vi "Initial Values-Compare-STRING.vi"(5 "Function (Add)":T1=enum."Add", 7 "Current values":string[](array[string]), 8 "error in (no error)":errorcluster, 9 "Keys Array":T4, 10 "Section name":string, 11 "User profile ini file ref":T5) -> (0 "error out":errorcluster, 1 "Keys of changed parameters":T3, 2 "Changed parameters info":T2[](array[typedef]), 3 "User profile ini file ref":T5, 4 "Changes exist":bool)   [LabVIEW 2017]
uses:
  Typedefs/Ini file interface (String).ctl
  <vilib>/Utility/config.llb/Config Data RefNum.ctl
  User Interface/User profiles code/Typedefs/Changes info cluster-STRING.ctl
  User Interface/User profiles code/Typedefs/Changed parameter cluster.ctl
  User Interface/User profiles code/Typedefs/Comparison states.ctl
  <userlib>/_OpenG.lib/array/array.llb/Search 1D Array (Boolean)__ogtk.vi
  <userlib>/_OpenG.lib/array/array.llb/Index 1D Array Elements (String)__ogtk.vi
  <userlib>/_OpenG.lib/array/array.llb/Index 1D Array Elements (Variant)__ogtk.vi
  <vilib>/Utility/config.llb/NI_LVConfig.lvlib
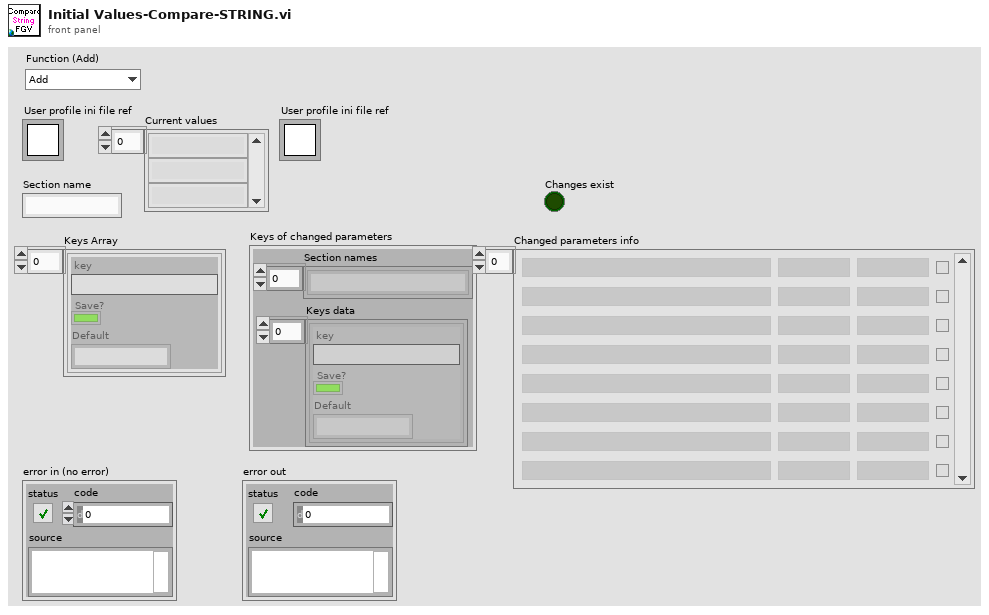
[diagram p1: front panel]
types:
  T1 = typedef "Comparison states.ctl" = enum16{"Init.", "Add", "Read"}
  T2 = typedef "Changed parameter cluster.ctl" = cluster{"Name":string, "Old value":string, "New value":string, "Save":bool}
  T3 = typedef "Changes info cluster-STRING.ctl" = cluster{"Section names":string[], "Keys data":T4}
  T4 = typedef "Ini file interface (String).ctl" = cluster{"key":string, "Save?":bool, "Default":string}[]
  T5 = typedef "NI_LVConfig.lvlib/Config Data RefNum.ctl" = refnum<k1>
  T6 = cluster{"key":string, "Save?":bool, "Default":string}
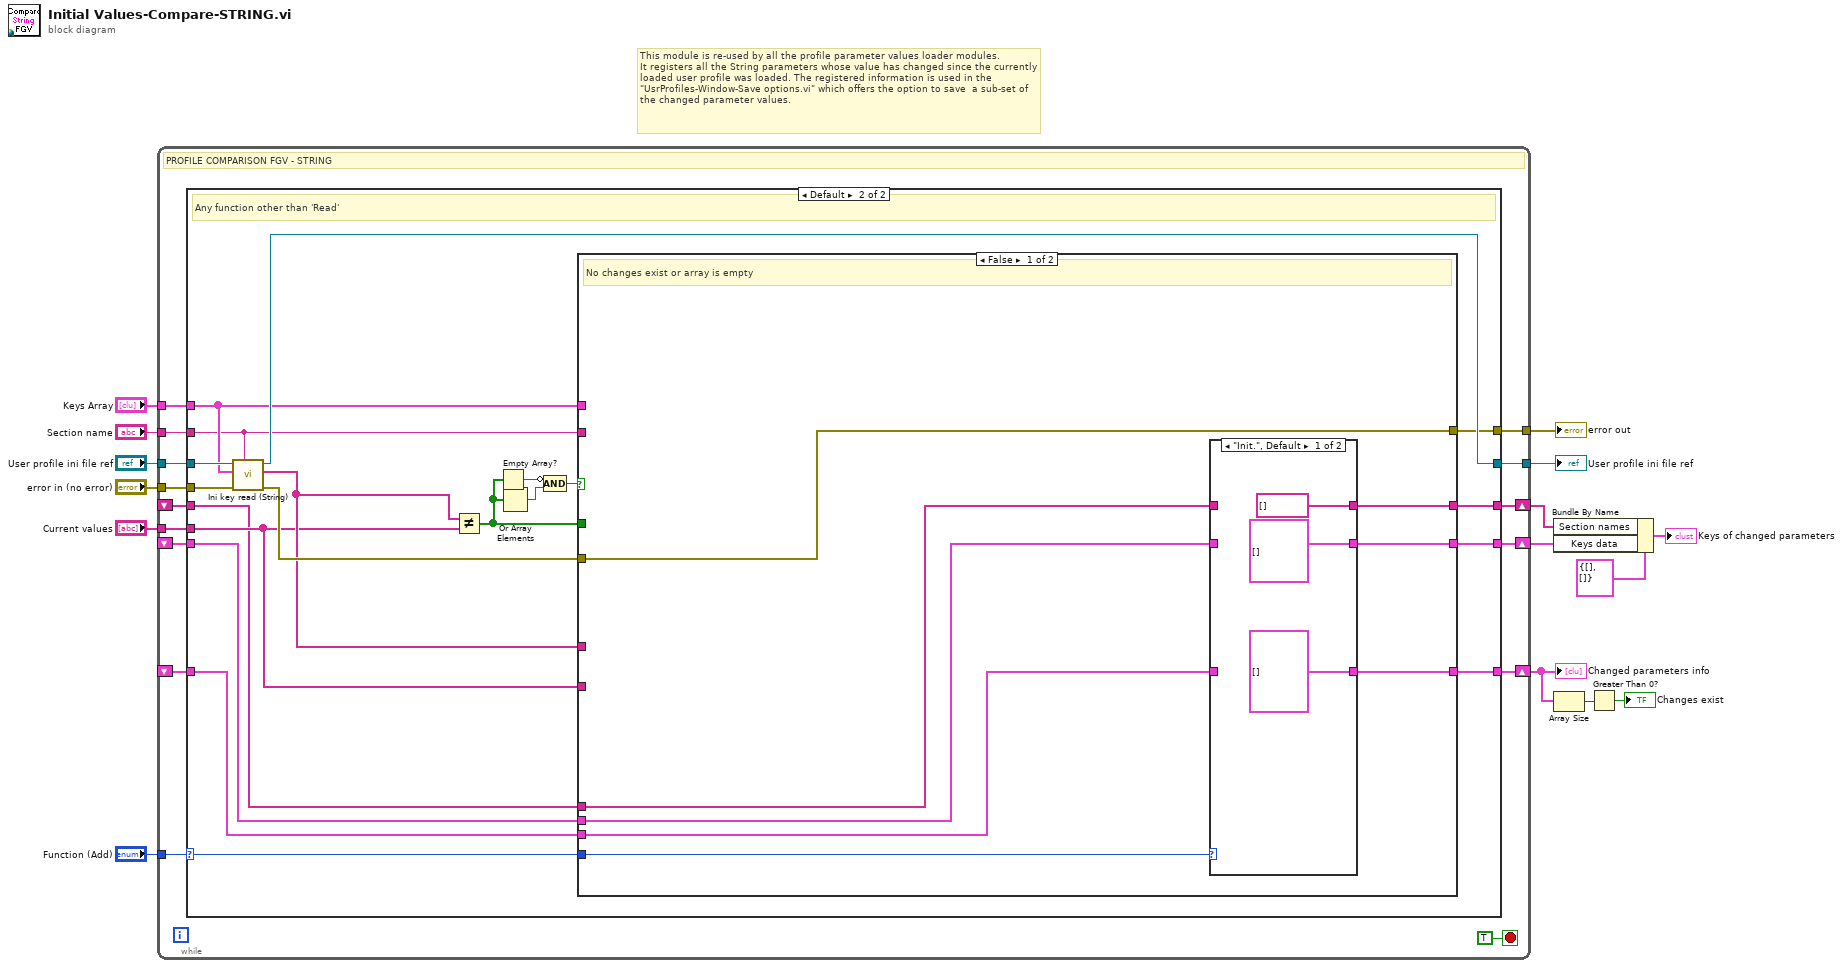
[diagram p0: block diagram]
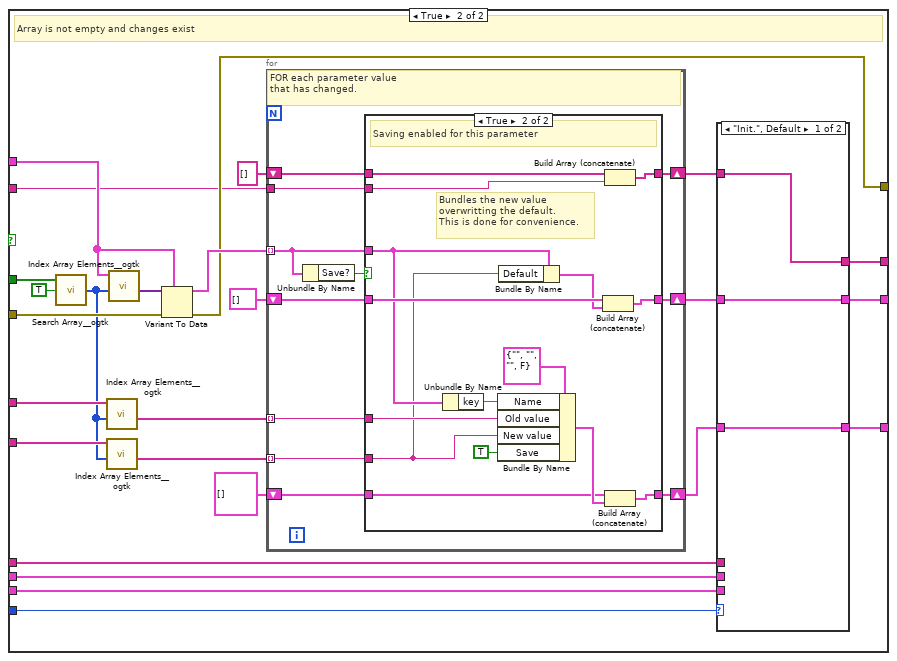
[diagram p4: hidden frame]
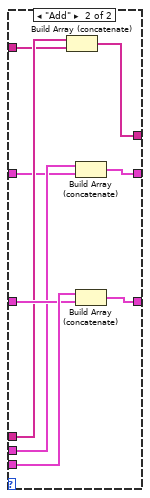
[diagram p5: hidden frame]
diagram:
  # "This module is re-used by all the profile parameter values loader modules.\nIt registers all the String parameters whose value has changed since the currently loaded user profile was loaded. The registered information is used in the \"UsrProfiles-Window-Save options.vi\" which offers the option to save  a sub-set of the changed parameter values."
  n1 = while {
    tunnel: "Section name" -> [w30]
    tunnel: "error in (no error)" -> [w29]
    tunnel: [w28] -> w13
    tunnel: "User profile ini file ref" -> [w27]
    tunnel: "Keys Array" -> [w20]
    tunnel: "Current values" -> [w19]
    tunnel: [w25] -> w9
    shift-right: [w21] -> w2
    shift-left: _ -> [w23]
    shift-right: [w24] -> w5
    shift-left: _ -> [w22]
    tunnel: "Function (Add)" -> [w18]
    shift-right: [w17] -> w1
    shift-left: _ -> [w16]
    stop <- TRUE stop-if-true
    # "PROFILE COMPARISON FGV - STRING"
    n2 = case shown="Default" w18 {
      selector: w18 -> [_ w39]
      tunnel: w30 -> [_ w38]
      tunnel: w29 -> [w35 w55]
      tunnel: [w34 w54] -> w28
      tunnel: w27 -> [w34 w53]
      tunnel: [w35 w51] -> w25
      tunnel: [w32 w50] -> w24
      tunnel: w23 -> [w33 w49]
      tunnel: w22 -> [w32 w48]
      tunnel: [w33 w44] -> w21
      tunnel: w20 -> [_ w43]
      tunnel: w19 -> [_ w41]
      tunnel: [w31 w37] -> w17
      tunnel: w16 -> [w31 w36]
      frame "Read" {
        # "The selected function is 'Read'"
      }
      frame Default {
        # "Any function other than 'Read'"
        n3 = call "Ini key read (String).vi"("Section name"=w38, "error in (no error)"=w55, "Keys setup"=w43, "Ini file ref in"=w53) -> ("error out"=w52:errorcluster, "Value read/used"=w42:string[], "Ini file ref"=w54:T5)  [unwired: 5 in]
        n4 = Not Equal?(x=w42, y=w41) -> (x != y?=w40:bool[])
        n5 = Empty Array?(array=w40) -> (empty?=w47:bool)
        n6 = Or Array Elements(Boolean array=w40) -> (logical OR=w46:bool)
        n7 = Compound Arithmetic op=AND(invert w47, w46) -> (w45:bool)
        n8 = case shown="False" w45 {
          tunnel: w43 -> [_ w95]
          tunnel: w41 -> [_ w94]
          tunnel: w40 -> [_ w93]
          tunnel: w52 -> [w63 w90]
          tunnel: w42 -> [_ w89]
          tunnel: w39 -> [w59 w84]
          tunnel: [w63 w78] -> w51
          tunnel: [w60 w81] -> w50
          tunnel: w49 -> [w62 w80]
          tunnel: w48 -> [w61 w79]
          tunnel: [w56 w76] -> w44
          tunnel: w38 -> [_ w74]
          tunnel: [w57 w71] -> w37
          tunnel: w36 -> [w58 w70]
          frame False {
            # "No changes exist or array is empty"
            n9 = case shown="\"Init.\", Default" w59 {
              tunnel: w62 -> [_ w68]
              tunnel: w61 -> [_ w69]
              tunnel: [T2[] [] ("Changed parameters info") w69] -> w60
              tunnel: [T4 [] ("Keys of changed parameters") w68] -> w56
              tunnel: [string[] [] w67] -> w57
              tunnel: w58 -> [_ w67]
              frame "Init.", Default {
              }
              frame "Add" {
              }
            }
          }
          frame True {
            # "Array is not empty and changes exist"
            n10 = call-poly <userlib>:"Search Array__ogtk.vi"("Array"=w93, "Element Data"=TRUE) -> ("Indices of Elements"=w87:i32[])  [unwired: 7 in]
            n11 = call-poly <userlib>:"Index Array Elements__ogtk.vi"("indices"=w87, "array"=w89) -> ("elements"=w88:string[])  [unwired: 9 in]
            n12 = call-poly <userlib>:"Index Array Elements__ogtk.vi"("indices"=w87, "array"=w94) -> ("elements"=w86:string[])  [unwired: 9 in]
            n13 = call-poly <userlib>:"Index Array Elements__ogtk.vi"("indices"=w87, "array"=w95) -> ("elements"=w91:variant[])  [unwired: 9 in]
            n14 = Variant To Data(error in=w90, type=w95, Variant=w91) -> (data=w85:T4, error out=w78:errorcluster)
            n15 = for {
              tunnel: w88 -> [w118] mode=indexing
              tunnel: w86 -> [w117] mode=indexing
              tunnel: w85 -> [w114] mode=indexing
              shift-right: [w115] -> w83
              shift-left: T4 [] ("Keys of changed parameters") -> [w116]
              shift-right: [w113] -> w82
              shift-left: T2[] [] -> [w112]
              tunnel: w74 -> [w110]
              shift-right: [w109] -> w72
              shift-left: string[] [] -> [w108]
              # "FOR each parameter value\nthat has changed."
              n16 = Unbundle By Name(w114) -> ("Save?"=w111:bool)
              n17 = case shown="True" w111 {
                tunnel: w118 -> [_ w126]
                tunnel: w117 -> [_ w125]
                tunnel: w116 -> [w121 w133]
                tunnel: [w121 w131] -> w115
                tunnel: w114 -> [_ w130]
                tunnel: [w120 w128] -> w113
                tunnel: w112 -> [w120 w127]
                tunnel: w110 -> [_ w124]
                tunnel: [w119 w123] -> w109
                tunnel: w108 -> [w119 w122]
                frame False {
                  # "Saving disabled for this parameter"
                }
                frame True {
                  # "Bundles the new value\noverwritting the default.\nThis is done for convenience."
                  # "Saving enabled for this parameter"
                  n18 = Unbundle By Name(w130) -> ("key"=w134:string)
                  n19 = Bundle By Name(cluster=T2 {"Name"="", "Old value"="", "New value"="", "Save"=FALSE} ("Cluster"), "Name"=w134, "Old value"=w126, "New value"=w125, "Save"=TRUE) -> (w129:T2)
                  n20 = Bundle By Name(cluster=w130, "Default"=w125) -> (w132:T6)
                  n21 = Build Array (concatenate)(w133, w132) -> (w131:T4)
                  n22 = Build Array (concatenate)(w122, w124) -> (w123:string[])
                  n23 = Build Array (concatenate)(w127, w129) -> (w128:T2[])
                }
              }
            }
            n24 = case shown="\"Init.\", Default" w84 {
              tunnel: w83 -> [w97 w99]
              tunnel: w82 -> [w98 w103]
              tunnel: [w98 w107] -> w81
              tunnel: w80 -> [_ w102]
              tunnel: w79 -> [_ w104]
              tunnel: [w97 w106] -> w76
              tunnel: w72 -> [w96 w100]
              tunnel: [w96 w105] -> w71
              tunnel: w70 -> [_ w101]
              frame "Init.", Default {
              }
              frame "Add" {
                n25 = Build Array (concatenate)(w101, w100) -> (w105:string[])
                n26 = Build Array (concatenate)(w102, w99) -> (w106:T4)
                n27 = Build Array (concatenate)(w104, w103) -> (w107:T2[])
              }
            }
          }
        }
      }
    }
  }
  "User profile ini file ref" <- w13
  "error out" <- w9
  "Changed parameters info" <- w5
  n28 = Bundle By Name(cluster=T3 {"Section names"=[], "Keys data"=[]} ("Keys of changed parameters"), "Section names"=w1, "Keys data"=w2) -> (→"Keys of changed parameters":T3)
  n29 = Array Size(array=w5) -> (size(s)=w7:i32)
  n30 = Greater Than 0?(x=w7) -> (x > 0?=→"Changes exist":bool)
